vi "GearTeleOp.vi"(10 "Buttons":bool[](array[boolean]), 11 "Robot":T1) -> ()   [LabVIEW 2015]
uses:
  Robot Type Def.ctl
  Framework/JoystickMappingNamesTypeDef.ctl
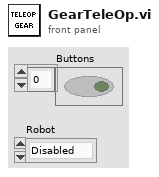
[diagram p1: front panel]
types:
  T1 = typedef "Robot Type Def.ctl" = enum32{"Disabled", "Ghost", "Casper", "Lofty", "Board", "RaceRobot", "Casper 2.0", "Excalibot 2.0"}
  T2 = typedef "JoystickMappingNamesTypeDef.ctl" = enum16{"Shoot Button", "Retrieve Button", "Arm Control", "High Gear", "Low Gear", "Enable PTO", "Disable PTO", "PortC Control", "PortC Up", "PortC Down", "Lift Control", "Drive VBus"}
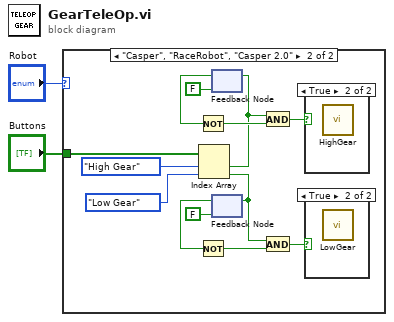
[diagram p0: block diagram]
diagram:
  n1 = case shown="\"Casper\", \"RaceRobot\", \"Casper 2.0\"" "Robot" {
    tunnel: "Buttons" -> [_ w15]
    frame Default {
    }
    frame "Casper", "RaceRobot", "Casper 2.0" {
      n2 = Index Array(array=w15, index #1=JoystickMappingNamesTypeDef."High Gear" ("Joystick Button Names"), index #2=JoystickMappingNamesTypeDef."Low Gear" ("Joystick Button Names")) -> (element #1=w5:bool, element #2=w3:bool)
      n3 = feedback #1(FALSE) -> (w12:bool)
      n4 = Not(x=w12) -> (.not. x?=w13:bool)
      n5 = feedback-in #1(w5) -> ()
      n6 = feedback #2(FALSE) -> (w8:bool)
      n7 = Not(x=w8) -> (.not. x?=w9:bool)
      n8 = feedback-in #2(w3) -> ()
      n9 = And(x=w5, y=w13) -> (x .and. y?=w11:bool)
      n10 = And(x=w3, y=w9) -> (x .and. y?=w7:bool)
      n11 = case shown="True" w11 {
        frame False {
        }
        frame True {
          n12 = call "HighGear.vi"() -> ()  [unwired: 11 in, 1 out]
        }
      }
      n13 = case shown="True" w7 {
        frame False {
        }
        frame True {
          n14 = call "LowGear.vi"() -> ()  [unwired: 12 in]
        }
      }
    }
  }
